vi "XY Sub VI.vi"(7 "Loop Count":i32, 8 "error in (no error)":errorcluster, 10 "XY State Machine In":T2, 11 "XY Params Input":T4={"Coordinates Input "={"X-axis (mm)"=0.0, "Y-axis (mm)"=0.0, "Y dist  target \nthreshold (mm)"=1.0, "X dist target\nthreshold (mm)"=0.0}, "X Axis Setpoint"={"X Frequency"=0.0, "X Accel"=0.0, "X Decel"=0.0, "X Speed (mm/s)"=0.0}, "Y Axis Setpoint"={"Y Max Speed \n(mm/s)"=0.0, "Y Max Accel\n(mm/s^2)"=0.0, "Y Max Decel \n(mm/s^2)"=0.0}} {"Coordinates Input"."X dist target\nthreshold (mm)" min=0.0; "Coordinates Input"."Y dist  target \nthreshold (mm)" min=0.0}) -> (0 "error out":errorcluster, 1 "Y Path Display":T5, 2 "Y Axis":T6(graph), 3 "X Axis":T6(graph), 4 "XY State Machine Out":T2)   [LabVIEW 2017]
uses:
  Motor Status Enum.ctl
  Coords Input Cluster.ctl
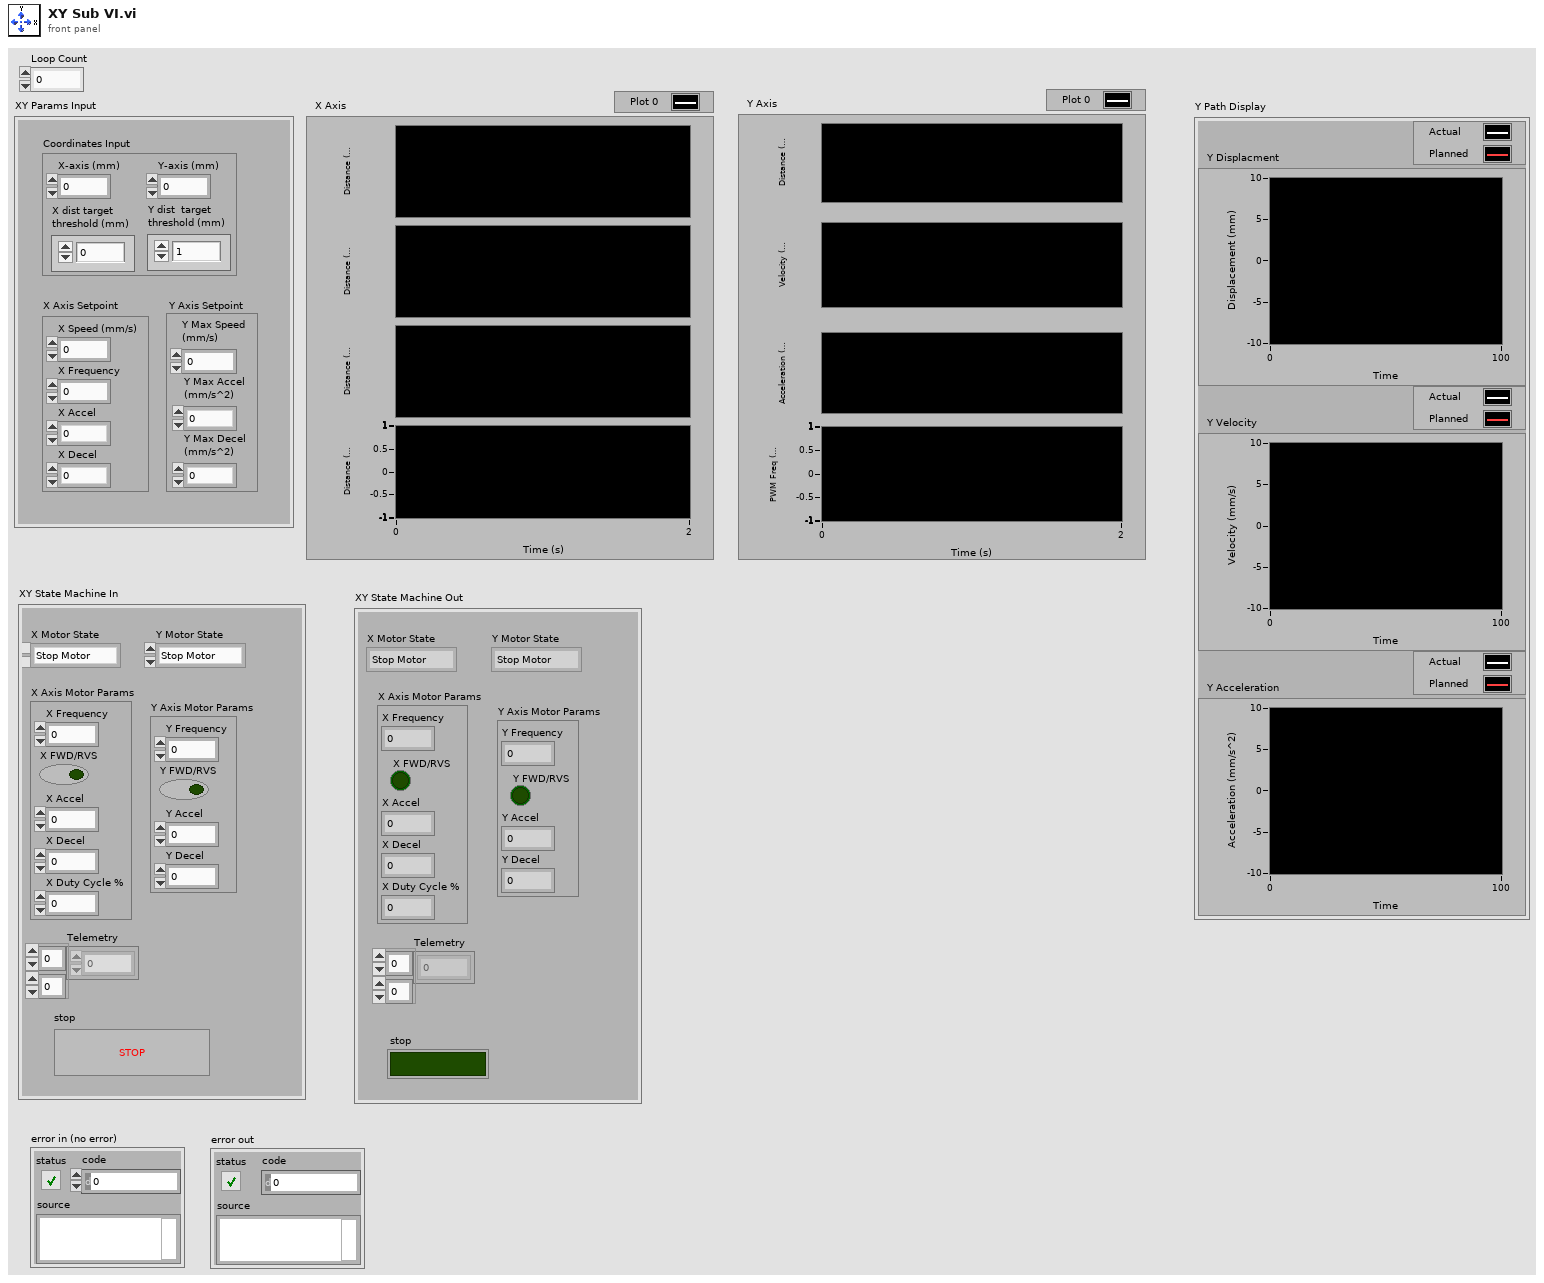
[diagram p1: front panel]
types:
  T1 = typedef "Motor Status Enum.ctl" = enum16{"Stop Motor", "Read Inputs", "Steady Speed", "Accelerate", "Decelerate"}
  T2 = cluster{"X Motor State":T1, "Y Motor State":T1, "X Axis Motor Params":cluster{"X Frequency":dbl, "X FWD/RVS":bool, "X Accel":dbl, "X Decel":dbl, "X Duty Cycle %":dbl}, "Telemetry":dbl[][], "stop":bool, "Y Axis Motor Params":cluster{"Y Frequency":dbl, "Y FWD/RVS":bool, "Y Accel":dbl, "Y Decel":dbl}}
  T3 = typedef "Coords Input Cluster.ctl" = cluster{"X-axis (mm)":dbl, "Y-axis (mm)":dbl, "Y dist  target \nthreshold (mm)":dbl, "X dist target\nthreshold (mm)":dbl}
  T4 = cluster{"Coordinates Input ":T3, "X Axis Setpoint":cluster{"X Frequency":dbl, "X Accel":dbl, "X Decel":dbl, "X Speed (mm/s)":dbl}, "Y Axis Setpoint":cluster{"Y Max Speed \n(mm/s)":dbl, "Y Max Accel\n(mm/s^2)":dbl, "Y Max Decel \n(mm/s^2)":dbl}}
  T5 = cluster{"Y Velocity":dbl[][], "Y Displacment":dbl[][], "Y Acceleration":dbl[][]}
  T6 = cluster{"X-axis distance":dbl, dbl, dbl, "X Frequency":dbl}
  T7 = cluster{"X Motor State in":T1, "Y Motor State in":T1, "X Axis Motor Params in":cluster{"X Frequency":dbl, "X FWD/RVS":bool, "X Accel":dbl, "X Decel":dbl, "X Duty Cycle %":dbl}, "Telemetry Input":dbl[][], "stop in":bool, "Y Axis Motor Params in":cluster{"Y Frequency":dbl, "Y FWD/RVS":bool, "Y Accel":dbl, "Y Decel":dbl}}
  T8 = cluster{"Target Coords (mm)":dbl, "Current Coords (mm)":dbl, "Max Speed (mm/s)":dbl, "Max Accel (mm/s^2)":dbl, "Max Decel (mm/s^2)":dbl}
  T9 = cluster{"Y Frequency":dbl, "Y FWD/RVS":bool, "Y Accel":dbl, "Y Decel":dbl}
  T10 = cluster{"Y Max Speed \n(mm/s)":dbl, "Y Max Accel\n(mm/s^2)":dbl, "Y Max Decel \n(mm/s^2)":dbl}
  T11 = cluster{"X Frequency":dbl, "X Accel":dbl, "X Decel":dbl, "X Speed (mm/s)":dbl}
  T12 = cluster{"X Frequency":dbl, "X FWD/RVS":bool, "X Accel":dbl, "X Decel":dbl, "X Duty Cycle %":dbl}
  T13 = typedef "Encoder Cluster.ctl" = cluster{"Y-axis rev count":dbl, "Y-axis distance":dbl, "X-axis rev count":dbl, "X-axis distance":dbl, "Y-axis direction":T14, "X-axis direction":T14, "X-counter val":i32, "Y-counter val":i32}
  T14 = typedef "Encoder Count Direction Enum.ctl" = enum16{"Counting Up", "Counting Down"}
  T15 = cluster{" Distance target (mm)":dbl, "Max Accel (mm/s^2)":dbl, "Max Decel (mm/s^2)":dbl, "Velocity Limit (mm/s) ":dbl, "Time step (s)":dbl}
  T16 = enum16{"800", "1600", "3200", "6400", "12800", "25600"}
  T17 = cluster{"Cruising Speed (mm/s)":dbl, "Crusing Time (s)":dbl, "Decel Time (s)":dbl, "Accel Time (s)":dbl, "Total Time (s)":dbl, "Accel Distance (mm)":dbl, "Decel Distance (mm)":dbl, "Crusing Distance (mm)":dbl}
  T18 = cluster{"X-axis distance":dbl, dbl, dbl, "X Duty Cycle %":dbl}
  T19 = cluster{"Y-axis distance":dbl, dbl, dbl, "Y Frequency":dbl}
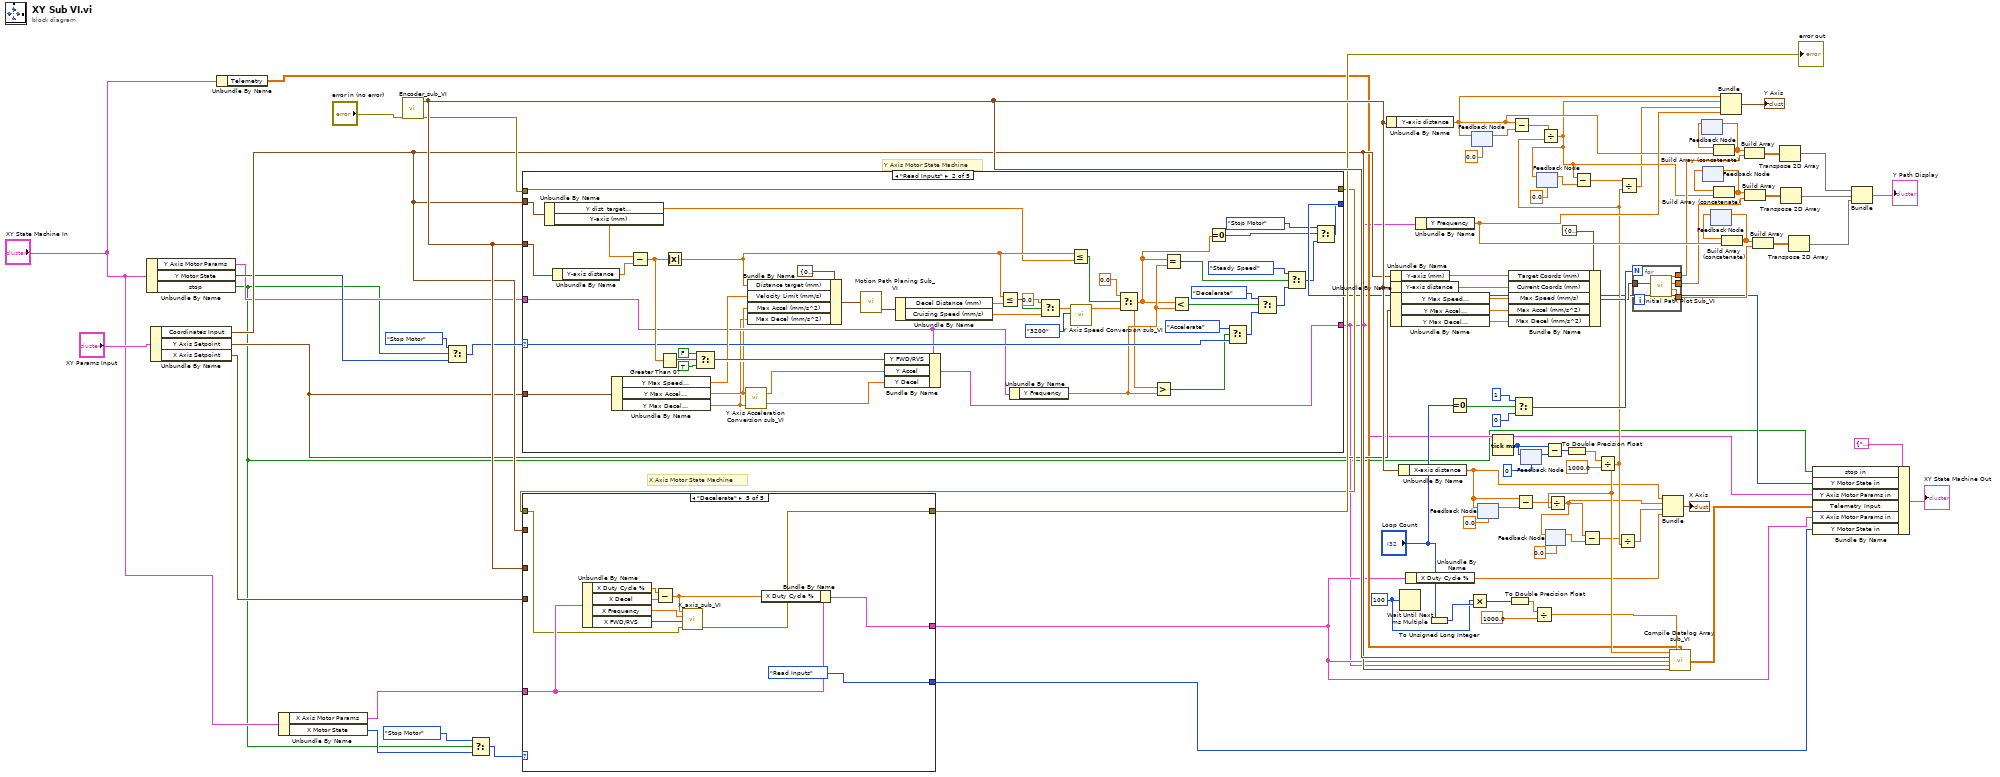
[diagram p0: block diagram]
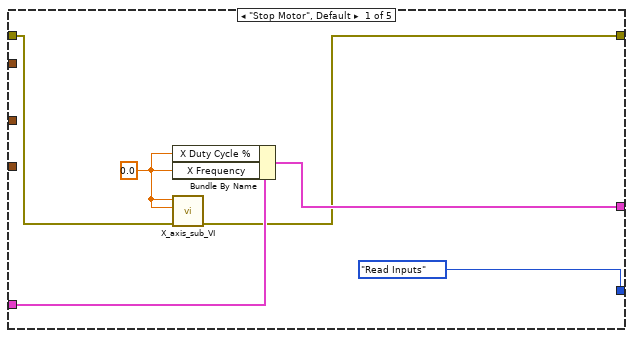
[diagram p2: hidden frame]
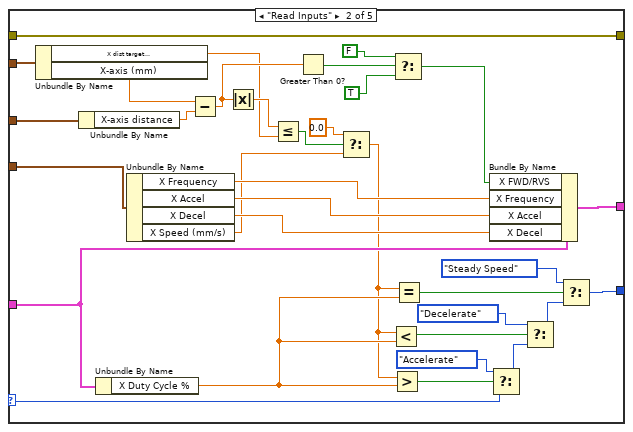
[diagram p3: hidden frame]
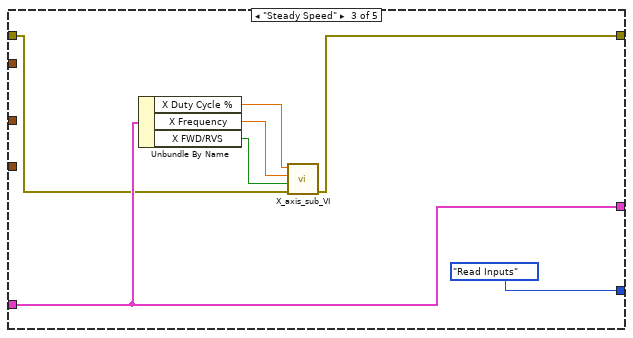
[diagram p4: hidden frame]
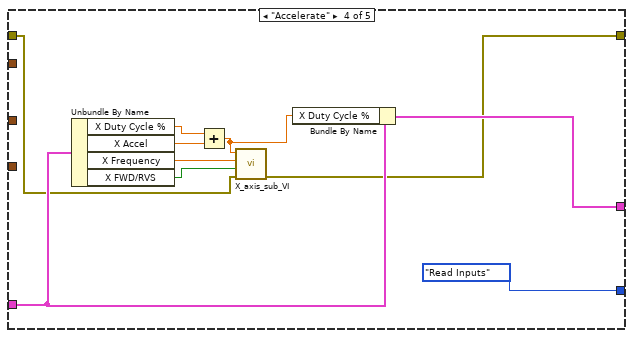
[diagram p5: hidden frame]
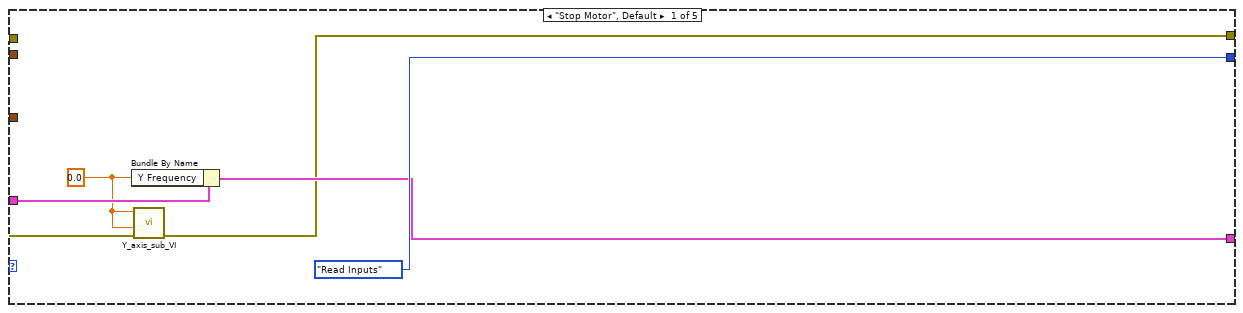
[diagram p6: hidden frame]
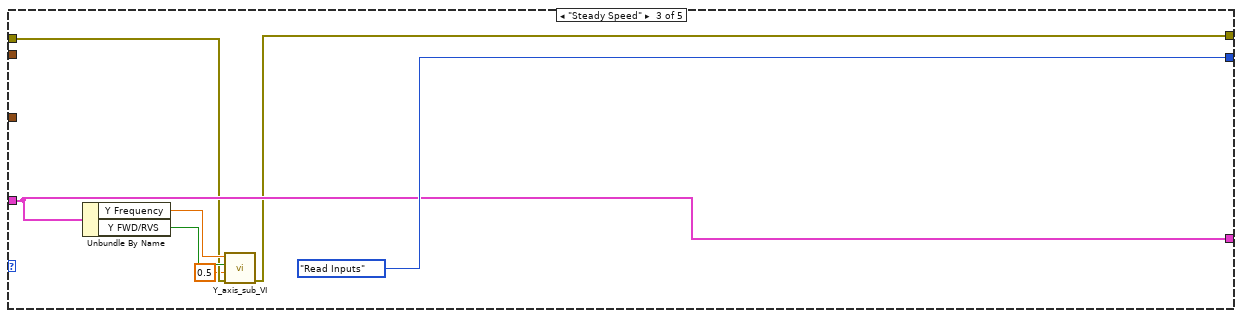
[diagram p7: hidden frame]
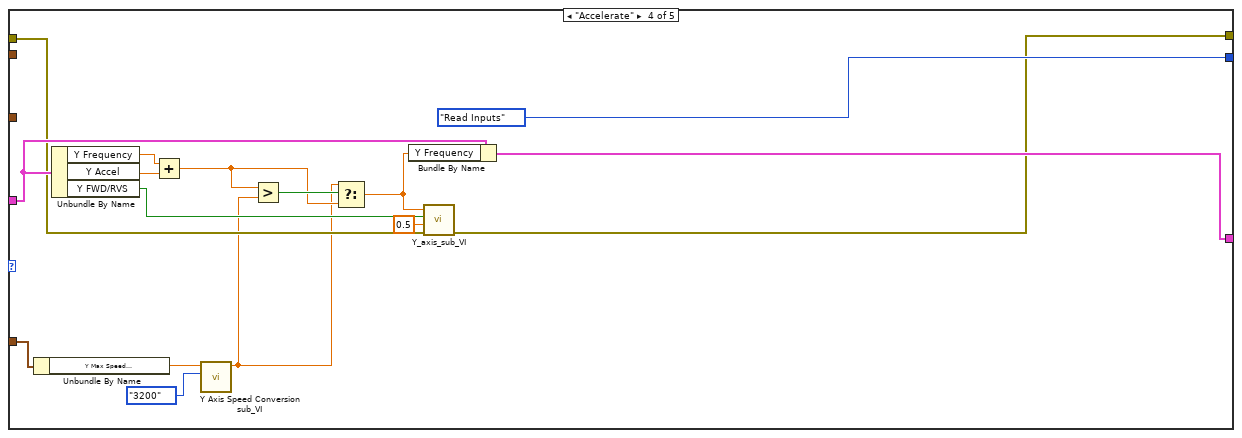
[diagram p8: hidden frame]
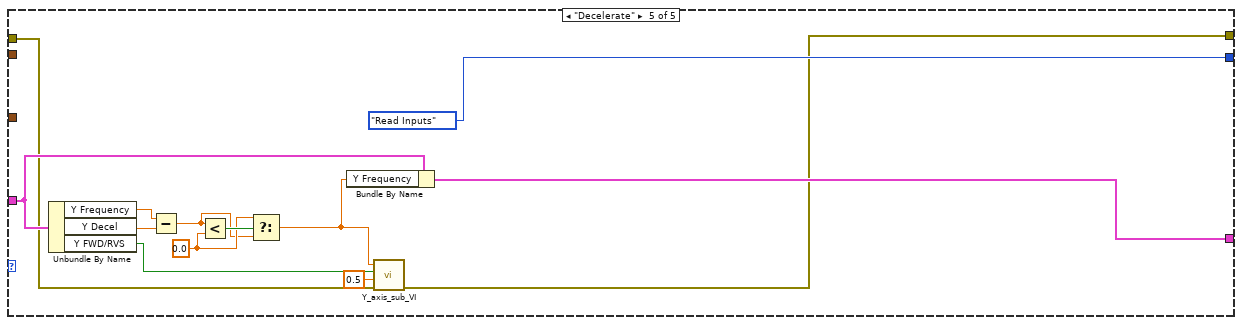
[diagram p9: hidden frame]
diagram:
  w38 = u32 100 ("milliseconds to wait")
  # "X Axis Motor State Machine"
  # "Y Axis Motor State Machine"
  n1 = Unbundle By Name("XY State Machine In") -> ("Y Axis Motor Params"=w10:T9, "Y Motor State"=w14:T1, "stop"=w3:bool)
  n2 = Unbundle By Name("XY Params Input") -> ("Coordinates Input"=w17:T3, "Y Axis Setpoint"=w15:T10, "X Axis Setpoint"=w16:T11)
  n3 = Unbundle By Name("XY State Machine In") -> ("Telemetry"=w13:dbl[][])
  n4 = Unbundle By Name("XY State Machine In") -> ("X Axis Motor Params"=w12:T12, "X Motor State"=w11:T1)
  n5 = call "Encoder_sub_VI.vi"("error in (no error)"="error in (no error)") -> ("error out"=w61:errorcluster, "Encoder Output"=w67:T13)  [unwired: 9 in]
  n6 = Select(t=Motor_Status_Enum."Stop Motor", s=w3, f=w14) -> (s? t:f=w26:T1)
  n7 = Select(t=Motor_Status_Enum."Stop Motor", s=w3, f=w11) -> (s? t:f=w29:T1)
  n8 = case shown="\"Read Inputs\"" w26 {
    selector: w26 -> [_ w114 _ _ _]
    tunnel: w10 -> [w96 w110 w147 w163 w175]
    tunnel: [Motor_Status_Enum."Read Inputs" w103 Motor_Status_Enum."Read Inputs" Motor_Status_Enum."Read Inputs" Motor_Status_Enum."Read Inputs"] -> w4
    tunnel: [w94 w101 w147 w162 w176] -> w5
    tunnel: w61 -> [w92 w116 w146 w160 w173]
    tunnel: [w93 w116 w145 w159 w174] -> w30
    tunnel: w67 -> [_ w118 _ _ _]
    tunnel: w17 -> [_ w117 _ _ _]
    tunnel: w15 -> [_ w102 _ w158 _]
    frame "Stop Motor", Default {
      w91 = 0.0 ("Y Frequency")
      n9 = Bundle By Name(cluster=w96, "Y Frequency"=w91) -> (w94:T9)
      n10 = call "Y_axis_sub_VI.vi"("error in (no error)"=w92, "Duty Cycle"=w91, "Frequency"=w91) -> ("error out"=w93:errorcluster)  [unwired: 8 in]
    }
    frame "Read Inputs" {
      n11 = Unbundle By Name(w117) -> ("Y dist  target \nthreshold (mm)"=w97:dbl, "Y-axis (mm)"=w129:dbl)
      n12 = Unbundle By Name(w118) -> ("Y-axis distance"=w128:dbl)
      n13 = Unbundle By Name(w102) -> ("Y Max Speed \n(mm/s)"=w115:dbl, "Y Max Accel\n(mm/s^2)"=w100:dbl, "Y Max Decel \n(mm/s^2)"=w99:dbl)
      n14 = Subtract(x=w129, y=w128) -> (x-y=w125:dbl)
      n15 = Greater Than 0?(x=w125) -> (x > 0?=w133:bool)
      n16 = Absolute Value(x=w125) -> (abs(x)=w108:dbl)
      n17 = Select(t=FALSE, s=w133, f=TRUE) -> (s? t:f=w134:bool)
      n18 = call "Y Axis Acceleration Conversion sub_VI.vi"("Deceleration (mm/s^2)"=w99, "Acceleration (mm/s^2)"=w100) -> ("Freq decrease per 0.1ms (Hz)"=w119:dbl, "Freq increase per 0.1ms (Hz)"=w120:dbl)
      n19 = Bundle By Name(cluster=T15 {" Distance target (mm)"=0.0, "Max Accel (mm/s^2)"=0.0, "Max Decel (mm/s^2)"=0.0, "Velocity Limit (mm/s) "=0.0, "Time step (s)"=0.0} ("Motion Planning Inputs"), "Distance target (mm)"=w108, "Velocity Limit (mm/s)"=w115, "Max Accel (mm/s^2)"=w100, "Max Decel (mm/s^2)"=w99) -> (w127:T15)
      n20 = call "Motion Path Planing Sub_VI.vi"("Motion Planning Inputs"=w127) -> ("Motion Planning Outputs"=w98:T17)  [unwired: 4 in, 2 out]
      n21 = Bundle By Name(cluster=w110, "Y FWD/RVS"=w134, "Y Accel"=w120, "Y Decel"=w119) -> (w101:T9)
      n22 = Unbundle By Name(w98) -> ("Decel Distance (mm)"=w124:dbl, "Cruising Speed (mm/s)"=w112:dbl)
      n23 = Less Or Equal?(x=w108, y=w124) -> (x <= y?=w123:bool)
      n24 = Unbundle By Name(w110) -> ("Y Frequency"=w111:dbl)
      n25 = Select(t=0.0, s=w123, f=w112) -> (s? t:f=w121:dbl)
      n26 = Less Or Equal?(x=w108, y=w97) -> (x <= y?=w109:bool)
      n27 = call "Y Axis Speed Conversion sub_VI.vi"("Microsteps per Rev"=T16."3200", "Setpoint\nSpeed (mm/s)"=w121) -> ("PWM Frequency"=w131:dbl)  [unwired: 9 in]
      n28 = Select(t=0.0, s=w109, f=w131) -> (s? t:f=w107:dbl)
      n29 = Greater?(x=w107, y=w111) -> (0:w113:bool)
      n30 = Equal?(x=w107, y=w111) -> (x = y?=w141:bool)
      n31 = Less?(x=w107, y=w111) -> (x < y?=w138:bool)
      n32 = Equal To 0?(x=w107) -> (x = 0?=w105:bool)
      n33 = Select(t=Motor_Status_Enum."Accelerate", s=w113, f=w114) -> (s? t:f=w140:T1)
      n34 = Select(t=Motor_Status_Enum."Decelerate", s=w138, f=w140) -> (s? t:f=w142:T1)
      n35 = Select(t=Motor_Status_Enum."Steady Speed", s=w141, f=w142) -> (s? t:f=w104:T1)
      n36 = Select(t=Motor_Status_Enum."Stop Motor", s=w105, f=w104) -> (s? t:f=w103:T1)
    }
    frame "Steady Speed" {
      n37 = Unbundle By Name(w147) -> ("Y Frequency"=w149:dbl, "Y FWD/RVS"=w150:bool)
      n38 = call "Y_axis_sub_VI.vi"("error in (no error)"=w146, "Duty Cycle"=0.5, "FWD/RVS"=w150, "Frequency"=w149) -> ("error out"=w145:errorcluster)  [unwired: 7 in]
    }
    frame "Accelerate" {
      n39 = Unbundle By Name(w158) -> ("Y Max Speed \n(mm/s)"=w153:dbl)
      n40 = Unbundle By Name(w163) -> ("Y Frequency"=w165:dbl, "Y Accel"=w166:dbl, "Y FWD/RVS"=w161:bool)
      n41 = Add(x=w165, y=w166) -> (x+y=w156:dbl)
      n42 = call "Y Axis Speed Conversion sub_VI.vi"("Microsteps per Rev"=T16."3200", "Setpoint\nSpeed (mm/s)"=w153) -> ("PWM Frequency"=w152:dbl)  [unwired: 9 in]
      n43 = Greater?(x=w156, y=w152) -> (0:w157:bool)
      n44 = Select(t=w152, s=w157, f=w156) -> (s? t:f=w155:dbl)
      n45 = Bundle By Name(cluster=w163, "Y Frequency"=w155) -> (w162:T9)
      n46 = call "Y_axis_sub_VI.vi"("error in (no error)"=w160, "Duty Cycle"=0.5, "FWD/RVS"=w161, "Frequency"=w155) -> ("error out"=w159:errorcluster)  [unwired: 7 in]
    }
    frame "Decelerate" {
      w170 = 0.0 ("y")
      n47 = Unbundle By Name(w175) -> ("Y Frequency"=w179:dbl, "Y Decel"=w178:dbl, "Y FWD/RVS"=w172:bool)
      n48 = Subtract(x=w179, y=w178) -> (x-y=w169:dbl)
      n49 = Less?(x=w169, y=w170) -> (x < y?=w171:bool)
      n50 = Select(t=w170, s=w171, f=w169) -> (s? t:f=w168:dbl)
      n51 = Bundle By Name(cluster=w175, "Y Frequency"=w168) -> (w176:T9)
      n52 = call "Y_axis_sub_VI.vi"("error in (no error)"=w173, "Duty Cycle"=0.5, "FWD/RVS"=w172, "Frequency"=w168) -> ("error out"=w174:errorcluster)  [unwired: 7 in]
    }
  }
  n53 = case shown="\"Decelerate\"" w29 {
    selector: w29 -> [_ w206 _ _ _]
    tunnel: [Motor_Status_Enum."Read Inputs" w200 Motor_Status_Enum."Read Inputs" Motor_Status_Enum."Read Inputs" Motor_Status_Enum."Read Inputs"] -> w6
    tunnel: [w182 w205 w222 w230 w239] -> w7
    tunnel: w12 -> [w183 w204 w222 w229 w238]
    tunnel: w30 -> [w181 w203 w220 w228 w237]
    tunnel: [w180 w203 w219 w227 w236] -> w31
    tunnel: w67 -> [_ w202 _ _ _]
    tunnel: w17 -> [_ w201 _ _ _]
    tunnel: w16 -> [_ w186 _ _ _]
    frame "Stop Motor", Default {
      w185 = 0.0 ("Y Frequency")
      n54 = Bundle By Name(cluster=w183, "X Duty Cycle %"=w185, "X Frequency"=w185) -> (w182:T12)
      n55 = call "X_axis_sub_VI.vi"("error in (no error)"=w181, "Frequency"=w185, "Duty Cycle %"=w185) -> ("error out"=w180:errorcluster)  [unwired: 8 in]
    }
    frame "Read Inputs" {
      n56 = Unbundle By Name(w201) -> ("X dist target\nthreshold (mm)"=w187:dbl, "X-axis (mm)"=w192:dbl)
      n57 = Unbundle By Name(w202) -> ("X-axis distance"=w191:dbl)
      n58 = Unbundle By Name(w204) -> ("X Duty Cycle %"=w217:dbl)
      n59 = Unbundle By Name(w186) -> ("X Frequency"=w209:dbl, "X Accel"=w207:dbl, "X Decel"=w208:dbl, "X Speed (mm/s)"=w196:dbl)
      n60 = Subtract(x=w192, y=w191) -> (x-y=w189:dbl)
      n61 = Absolute Value(x=w189) -> (abs(x)=w188:dbl)
      n62 = Less Or Equal?(x=w188, y=w187) -> (x <= y?=w190:bool)
      n63 = Greater Than 0?(x=w189) -> (x > 0?=w198:bool)
      n64 = Select(t=0.0, s=w190, f=w196) -> (s? t:f=w195:dbl)
      n65 = Less?(x=w195, y=w217) -> (x < y?=w212:bool)
      n66 = Greater?(x=w195, y=w217) -> (0:w210:bool)
      n67 = Select(t=FALSE, s=w198, f=TRUE) -> (s? t:f=w193:bool)
      n68 = Equal?(x=w195, y=w217) -> (x = y?=w216:bool)
      n69 = Bundle By Name(cluster=w204, "X FWD/RVS"=w193, "X Frequency"=w209, "X Accel"=w207, "X Decel"=w208) -> (w205:T12)
      n70 = Select(t=Motor_Status_Enum."Accelerate", s=w210, f=w206) -> (s? t:f=w214:T1)
      n71 = Select(t=Motor_Status_Enum."Decelerate", s=w212, f=w214) -> (s? t:f=w215:T1)
      n72 = Select(t=Motor_Status_Enum."Steady Speed", s=w216, f=w215) -> (s? t:f=w200:T1)
    }
    frame "Steady Speed" {
      n73 = Unbundle By Name(w222) -> ("X Duty Cycle %"=w224:dbl, "X Frequency"=w223:dbl, "X FWD/RVS"=w225:bool)
      n74 = call "X_axis_sub_VI.vi"("error in (no error)"=w220, "FWD/RVS"=w225, "Frequency"=w223, "Duty Cycle %"=w224) -> ("error out"=w219:errorcluster)  [unwired: 7 in]
    }
    frame "Accelerate" {
      n75 = Unbundle By Name(w229) -> ("X Duty Cycle %"=w232:dbl, "X Accel"=w233:dbl, "X Frequency"=w234:dbl, "X FWD/RVS"=w226:bool)
      n76 = Add(x=w232, y=w233) -> (x+y=w235:dbl)
      n77 = call "X_axis_sub_VI.vi"("error in (no error)"=w228, "FWD/RVS"=w226, "Frequency"=w234, "Duty Cycle %"=w235) -> ("error out"=w227:errorcluster)  [unwired: 7 in]
      n78 = Bundle By Name(cluster=w229, "X Duty Cycle %"=w235) -> (w230:T12)
    }
    frame "Decelerate" {
      n79 = Unbundle By Name(w238) -> ("X Duty Cycle %"=w241:dbl, "X Decel"=w242:dbl, "X Frequency"=w243:dbl, "X FWD/RVS"=w245:bool)
      n80 = Subtract(x=w241, y=w242) -> (x-y=w244:dbl)
      n81 = call "X_axis_sub_VI.vi"("error in (no error)"=w237, "FWD/RVS"=w245, "Frequency"=w243, "Duty Cycle %"=w244) -> ("error out"=w236:errorcluster)  [unwired: 7 in]
      n82 = Bundle By Name(cluster=w238, "X Duty Cycle %"=w244) -> (w239:T12)
    }
  }
  "error out" <- w31
  n83 = Unbundle By Name(w67) -> ("Y-axis distance"=w83:dbl)
  n84 = Unbundle By Name(w17) -> ("Y-axis (mm)"=w68:dbl)
  n85 = Unbundle By Name(w67) -> ("Y-axis distance"=w69:dbl)
  n86 = Unbundle By Name(w15) -> ("Y Max Speed \n(mm/s)"=w64:dbl, "Y Max Accel\n(mm/s^2)"=w65:dbl, "Y Max Decel \n(mm/s^2)"=w66:dbl)
  n87 = Unbundle By Name(w67) -> ("X-axis distance"=w58:dbl)
  n88 = Wait Until Next ms Multiple(millisecond multiple=w38) -> ()  [unwired: 1 out]
  n89 = Unbundle By Name(w7) -> ("X Duty Cycle %"=w43:dbl)
  n90 = Unbundle By Name(w5) -> ("Y Frequency"=w89:dbl)
  n91 = To Unsigned Long Integer(number="Loop Count") -> (unsigned 32bit integer=w39:u32)
  n92 = Equal To 0?(x="Loop Count") -> (x = 0?=w70:bool)
  n93 = Multiply(x=w38, y=w39) -> (x*y=w40:u32)
  n94 = feedback #1(0.0) -> (w45:dbl)
  n95 = feedback-in #1(w83) -> ()
  n96 = feedback #2(0.0) -> (w51:dbl)
  n97 = feedback-in #2(w58) -> ()
  n98 = Tick Count (ms)() -> (millisecond timer value=w36:u32)
  n99 = Bundle By Name(cluster=T8 {"Target Coords (mm)"=0.0, "Current Coords (mm)"=0.0, "Max Speed (mm/s)"=0.0, "Max Accel (mm/s^2)"=0.0, "Max Decel (mm/s^2)"=0.0} ("Motion Inputs"), "Target Coords (mm)"=w68, "Current Coords (mm)"=w69, "Max Speed (mm/s)"=w64, "Max Accel (mm/s^2)"=w65, "Max Decel (mm/s^2)"=w66) -> (w63:T8)
  n100 = To Double Precision Float(number=w40) -> (double precision float=w41:dbl)
  n101 = Subtract(x=w83, y=w45) -> (x-y=w46:dbl)
  n102 = Select(t=1, s=w70, f=0) -> (s? t:f=w71:i32)
  n103 = Subtract(x=w58, y=w51) -> (x-y=w52:dbl)
  n104 = feedback #3(u32 0) -> (w37:u32)
  n105 = feedback-in #3(w36) -> ()
  n106 = Divide(x=w41, y=1000.0) -> (x/y=w42:dbl)
  n107 = feedback #4(0.0) -> (w48:dbl)
  n108 = Subtract(x=w36, y=w37) -> (x-y=w33:u32)
  n109 = feedback #5(0.0) -> (w54:dbl)
  n110 = To Double Precision Float(number=w33) -> (double precision float=w35:dbl)
  n111 = Divide(x=w35, y=1000.0) -> (x/y=w59:dbl)
  n112 = Divide(x=w46, y=w59) -> (x/y=w76:dbl)
  n113 = feedback-in #4(w76) -> ()
  n114 = Divide(x=w52, y=w59) -> (x/y=w56:dbl)
  n115 = feedback-in #5(w56) -> ()
  n116 = Subtract(x=w76, y=w48) -> (x-y=w49:dbl)
  n117 = Subtract(x=w56, y=w54) -> (x-y=w55:dbl)
  n118 = Divide(x=w55, y=w59) -> (x/y=w57:dbl)
  n119 = Divide(x=w49, y=w59) -> (x/y=w74:dbl)
  n120 = for {
    N: w71 -> [_]
    tunnel: w63 -> [w249]
    tunnel: [w248] -> w78
    tunnel: [w247] -> w84
    tunnel: [w246] -> w88
    n121 = call "Initial Path Plot Sub_VI.vi"("Motion Inputs"=w249) -> ("Accel Array"=w246:dbl[], "Velocity Array"=w248:dbl[], "Displacement Array"=w247:dbl[])  [unwired: 3 in, 5 out]
  }
  n122 = Bundle("X-axis distance"=w58, w56, w57, "X Duty Cycle %"=w43) -> (→"X Axis":T18)  [unwired: 1 in]
  n123 = call "Compile Datalog Array sub_VI.vi"("Loop Runtime (s)"=w59, "Total Runtime (s)"=w42, "Initialised Array"=w13, "Encoder Output"=w67, "X Axis Motor Params"=w7, "Y Axis Motor Params"=w5, "Coordinates Input"=w17) -> ("Data Array"=w8:dbl[][])  [unwired: 8 in]
  n124 = feedback #6() -> (w82:dbl[])  [unwired: 1 in]
  n125 = feedback #7() -> (w75:dbl[])  [unwired: 1 in]
  n126 = feedback #8() -> (w87:dbl[])  [unwired: 1 in]
  n127 = Build Array (concatenate)(w82, w83) -> (w81:dbl[])
  n128 = feedback-in #6(w81) -> ()
  n129 = Build Array (concatenate)(w75, w76) -> (w77:dbl[])
  n130 = feedback-in #7(w77) -> ()
  n131 = Bundle("Y-axis distance"=w83, w76, w74, "Y Frequency"=w89) -> (→"Y Axis":T19)  [unwired: 1 in]
  n132 = Build Array (concatenate)(w87, w89) -> (w86:dbl[])
  n133 = feedback-in #8(w86) -> ()
  n134 = Build Array(w81, w84) -> (w80:dbl[][])
  n135 = Build Array(w77, w78) -> (w79:dbl[][])
  n136 = Build Array(w86, w88) -> (w85:dbl[][])
  n137 = Transpose 2D Array(2D array=w80) -> (transposed array=w23:dbl[][])
  n138 = Transpose 2D Array(2D array=w79) -> (transposed array=w22:dbl[][])
  n139 = Transpose 2D Array(2D array=w85) -> (transposed array=w21:dbl[][])
  n140 = Bundle By Name(cluster=T7 {"X Motor State in"=enum."Stop Motor", "Y Motor State in"=enum."Stop Motor", "X Axis Motor Params in"={"X Frequency"=0.0, "X FWD/RVS"=FALSE, "X Accel"=0.0, "X Decel"=0.0, "X Duty Cycle %"=0.0}, "Telemetry Input"=[], "stop in"=FALSE, "Y Axis Motor Params in"={"Y Frequency"=0.0, "Y FWD/RVS"=FALSE, "Y Accel"=0.0, "Y Decel"=0.0}} ("XY State Machine In 3"), "stop in"=w3, "Y Motor State in"=w4, "Y Axis Motor Params in"=w5, "Telemetry Input"=w8, "X Axis Motor Params in"=w7, "Y Motor State in"=w6) -> (→"XY State Machine Out":T7)
  n141 = Bundle(w23, w22, w21) -> (→"Y Path Display":cluster{dbl[][], dbl[][], dbl[][]})  [unwired: 1 in]
